vi "Add Element.vi"(8 "error in (no error)":errorcluster caption="错误输入（无错误）", 10 "Element":variant, 11 "FIFO(DBL) 输入":refnum<class "FIFO(VAR).lvclass"> caption="DNL_LabVIEW Object in") -> (0 "error out":errorcluster caption="错误输出", 2 "Removed Element":variant, 3 "FIFO(DBL) 输出":refnum<class "FIFO(VAR).lvclass"> caption="DNL_LabVIEW Object out")   [LabVIEW 2012, in "FIFO(VAR).lvclass"]
uses:
  FIFO(VAR).lvclass
  FIFO(VAR).lvclass/FIFO(VAR).ctl
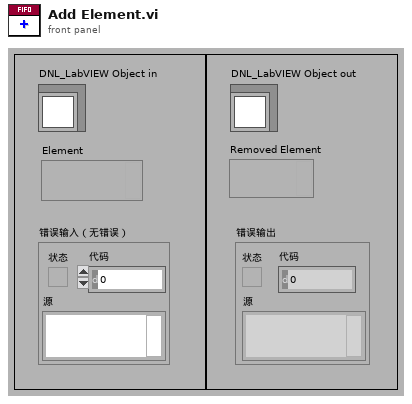
[diagram p1: front panel]
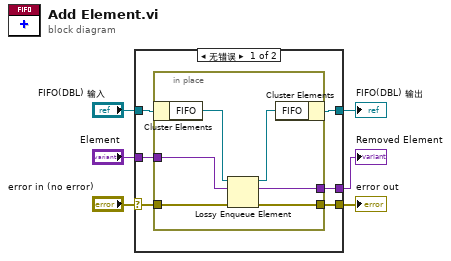
[diagram p0: block diagram]
diagram:
  n1 = case shown="无错误" "error in (no error)" {
    selector: "error in (no error)" -> [w10 w20]
    tunnel: [w9 w20] -> w5
    tunnel: [w11 w19] -> w3
    tunnel: "FIFO(DBL) 输入" -> [w12 w19]
    tunnel: "Element" -> [w8 _]
    tunnel: [w7 _] -> w1
    frame No Error {
      n2 = in-place {
        in-place-border: w10 -> [w16]
        in-place-border: [w15] -> w9
        in-place-border: w8 -> [w14]
        in-place-border: [w13] -> w7
        n3 = in-place-cluster #1(w12) -> ("FIFO"=w18:refnum<queue>)
        n4 = Lossy Enqueue Element(queue=w18, element=w14, error in (no error)=w16) -> (queue out=w17:refnum<queue>, overflow element=w13:variant, error out=w15:errorcluster)  [unwired: 1 out]
        n5 = in-place-cluster #1("FIFO"=w17) -> (w11:refnum<class "FIFO(VAR).lvclass">)
      }
    }
    frame Error {
    }
  }
  "error out" <- w5
  "FIFO(DBL) 输出" <- w3
  "Removed Element" <- w1
